vi "Class.SaveCtrls.Save.vi"(7 "Ignore Error":bool=TRUE, 8 "error in":errorcluster, 11 "CtrlStates In":refnum<class "Class.SaveCtrls.lvclass">) -> (0 "error out":errorcluster, 3 "CtrlStates":refnum<class "Class.SaveCtrls.lvclass">)   [LabVIEW 2024, in "EQMF.lvlib" / "Config Utils.lvlib" / "Class.SaveCtrls.lvclass"]
doc: "This VI is intended to be used at the application exit. This VI will obtain a list of control references and the data file path from the class data. That information was stored in the class by the InitLoadRestore.vi.\nIt will obtain all the control values form their references and will save the values to the file:\n<Module Data Dir>\\<Module Name>.dat\n\nINPUTS:\n<B>Ignore Errors</B> - If this is set to TRUE, any errors reading/writing to the file will eb ignored.\n\nOUTPUTS:\nNone\n\nERRORS: \nAn error will be reported if the file containing the control information cannot be opened."
uses:
  Class.SaveCtrls.lvclass
  Class.SaveCtrls.lvclass/Class.SaveCtrls.ctl
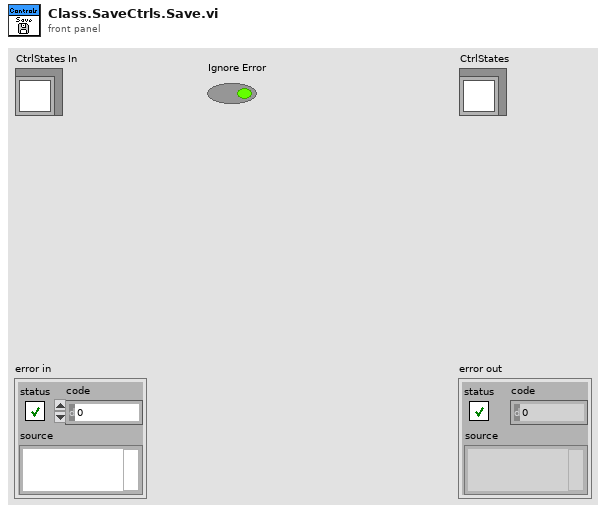
[diagram p1: front panel]
types:
  T1 = enum16{"open", "replace", "create", "open or create", "replace or create", "replace or create with confirmation"}
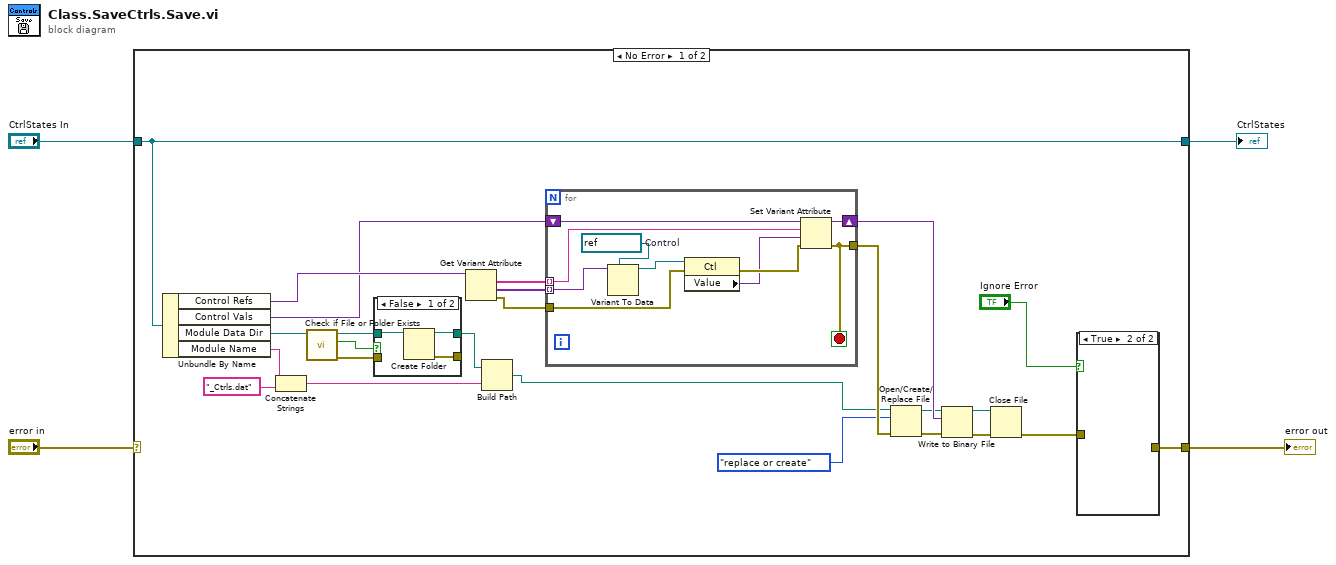
[diagram p0: block diagram]
diagram:
  n1 = case shown="No Error" "error in" {
    selector: "error in" -> [_ w46]
    tunnel: [w10 w46] -> w3
    tunnel: [w26 w45] -> w1
    tunnel: "CtrlStates In" -> [w26 w45]
    frame No Error {
      n2 = Unbundle By Name(w26) -> ("Control Refs"=w15:variant, "Control Vals"=w14:variant, "Module Data Dir"=w9:path, "Module Name"=w27:string)
      n3 = Concatenate Strings(w27, "_Ctrls.dat") -> (w29:string)
      n4 = call <vilib>:"Check if File or Folder Exists.vi"("path"=w9) -> ("error out"=w5:errorcluster, "file or folder exists?"=w8:bool, "dup path"=w7:path)  [unwired: 8 in]
      n5 = case shown="False" w8 {
        tunnel: w7 -> [w31 w33]
        tunnel: [w32 w33] -> w6
        tunnel: [w30 _] -> _
        tunnel: w5 -> [_ _]
        frame False {
          n6 = Create Folder(path (use dialog)=w31) -> (created path=w32:path, error out=w30:errorcluster)  [unwired: 2 in, 1 out]
        }
        frame True {
        }
      }
      n7 = Get Variant Attribute(Variant=w15) -> (names=w25:string[], values=w24:variant[], error out=w23:errorcluster)  [unwired: 3 in, 1 out]
      n8 = Build Path(base path=w6, name or relative path=w29) -> (appended path=w13:path)
      n9 = for {
        shift-right: [w43] -> w21
        shift-left: w14 -> [w44]
        tunnel: [w41] -> w22
        tunnel: w23 -> [w40]
        tunnel: w24 -> [w38] mode=indexing
        tunnel: w25 -> [w39] mode=indexing
        stop <- w41 stop-if-true
        w37 = refnum<vi> refnum  # Control
        n10 = Variant To Data(type=w37, Variant=w38) -> (data=w36:refnum<vi>)  [unwired: 1 in, 1 out]
        n11 = property class="Ctl"(reference=w36, error in=w40) -> (error out=w42:errorcluster, "Value"=w35:variant)  [unwired: 1 out]
        n12 = Set Variant Attribute(Variant=w44, name=w39, value=w35, error in=w42) -> (Variant out=w43:variant, error out=w41:errorcluster)  [unwired: 1 out]
      }
      n13 = Open/Create/Replace File(file path (use dialog)=w13, error in=w22, operation (0:open)=T1."replace or create") -> (refnum out=w16:refnum<file>, error out=w17:errorcluster)  [unwired: 3 in, 1 out]
      n14 = Write to Binary File(file (use dialog)=w16, data=w21, error in=w17) -> (refnum out=w18:refnum<file>, error out=w19:errorcluster)  [unwired: 3 in, 1 out]
      n15 = Close File(refnum=w18, error in=w19) -> (error out=w11:errorcluster)  [unwired: 1 out]
      n16 = case shown="True" "Ignore Error" {
        tunnel: w11 -> [w34 _]
        tunnel: [w34 _] -> w10
        frame False {
        }
        frame True {
        }
      }
    }
    frame Error {
    }
  }
  "error out" <- w3
  "CtrlStates" <- w1
